vi "Test Multiple Read Only Open.vi"(11 "Test Case In":refnum<class "Test Open Xml.lvclass">) -> (0 "error out":errorcluster, 3 "Test Case Out":refnum<class "Test Open Xml.lvclass">)   [LabVIEW 2020, in "Test Open Xml.lvclass"]
uses:
  Test Open Xml.lvclass
  Source/Open Xml.lvlib
  <vilib>/Astemes/LUnit/Test Case.lvclass
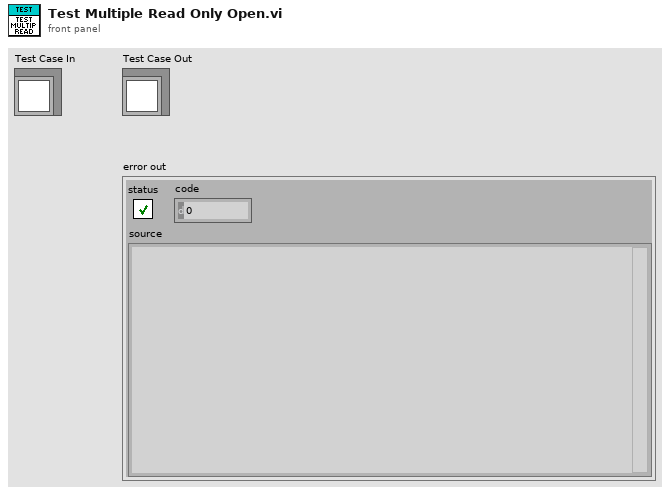
[diagram p1: front panel]
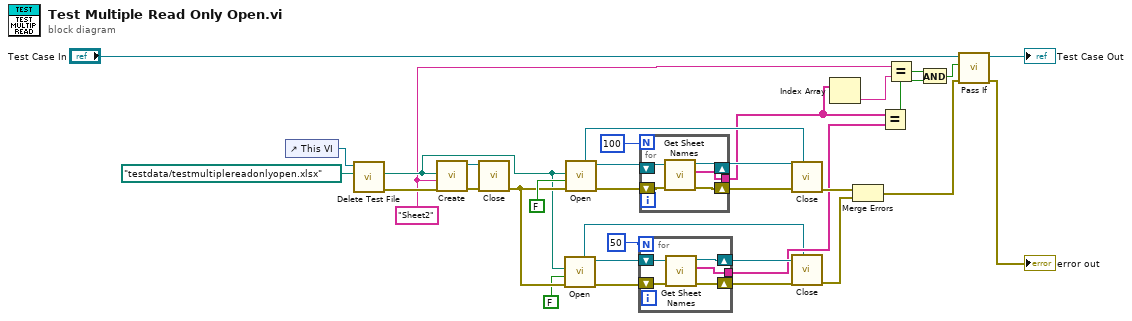
[diagram p0: block diagram]
diagram:
  w8 = "Sheet2" ("SheetName")
  n1 = control-ref of="This VI"() -> (w31:refnum<vi>)
  n2 = call "Delete Test File.vi"("name or relative path"=path "testdata/testmultiplereadonlyopen.xlsx", "VI in"=w31) -> ("error out"=w29:errorcluster, "deleted path"=w22:path)  [unwired: 8 in]
  n3 = call "Create.vi"("error in"=w29, "SheetName"=w8, "Path"=w22) -> ("error out"=w27:errorcluster, "SpreadsheetDoc"=w28:refnum<k24>)  [unwired: 7 in]
  n4 = call "Close.vi"("error in"=w27, "SpreadsheetDoc"=w28) -> ("error out"=w24:errorcluster)  [unwired: 9 in]
  n5 = call "Open.vi"("error in"=w24, "Editable (T)"=FALSE ("Editable"), "Path"=w22) -> ("error out"=w19:errorcluster, "SpreadsheetDoc"=w18:refnum<k24>, "Stream"=w1:refnum<k24>)  [unwired: 6 in]
  n6 = call "Open.vi"("error in"=w24, "Editable (T)"=FALSE ("Editable"), "Path"=w22) -> ("error out"=w21:errorcluster, "SpreadsheetDoc"=w20:refnum<k24>, "Stream"=w16:refnum<k24>)  [unwired: 6 in]
  n7 = for {
    N: 50 -> [_]
    shift-right: [w37] -> w17
    shift-left: w19 -> [w39]
    shift-right: [w36] -> w14
    shift-left: w18 -> [w38]
    tunnel: [w35] -> w10
    n8 = call "Get Sheet Names.vi"("error in"=w39, "SpreadsheetDoc in"=w38) -> ("error out"=w37:errorcluster, "Sheet Names"=w35:string[], "SpreadsheetDoc out"=w36:refnum<k24>)  [unwired: 7 in]
  }
  n9 = for {
    N: 100 -> [_]
    tunnel: [w40] -> w7
    shift-right: [w42] -> w15
    shift-left: w21 -> [w44]
    shift-right: [w41] -> w12
    shift-left: w20 -> [w43]
    n10 = call "Get Sheet Names.vi"("error in"=w44, "SpreadsheetDoc in"=w43) -> ("error out"=w42:errorcluster, "Sheet Names"=w40:string[], "SpreadsheetDoc out"=w41:refnum<k24>)  [unwired: 7 in]
  }
  n11 = call "Close.vi"("Stream"=w16, "error in"=w15, "SpreadsheetDoc"=w12) -> ("error out"=w26:errorcluster)  [unwired: 8 in]
  n12 = call "Close.vi"("Stream"=w1, "error in"=w17, "SpreadsheetDoc"=w14) -> ("error out"=w13:errorcluster)  [unwired: 8 in]
  n13 = Index Array(array=w7) -> (element=w6:string)  [unwired: 1 in]
  n14 = Merge Errors(w26, w13) -> (w3:errorcluster)
  n15 = Equal?(x=w7, y=w10) -> (x = y?=w4:bool)
  n16 = Equal?(x=w8, y=w6) -> (x = y?=w9:bool)
  n17 = And(x=w9, y=w4) -> (x .and. y?=w5:bool)
  n18 = call <vilib>:"Pass If.vi"("error in (no error)"=w3, "Pass?"=w5, "LUnit Test Case In"="Test Case In") -> ("error out"=→"error out":errorcluster, "LUnit Test Case Out"=→"Test Case Out":refnum<class "Test Open Xml.lvclass">)  [unwired: 7 in]
